vi "Force_Sensing2.vi"() -> ()   [LabVIEW 2014]
uses:
  <vilib>/Analysis/Matrix/Datatypes/RealMatrix.ctl
  <vilib>/Analysis/3filter.llb/Filter Passband Type.ctl
  <vilib>/Analysis/baseanly.llb/Real A x B.vi
  <vilib>/Analysis/_algsub.llb/Real PseudoInverse Matrix.vi
  <vilib>/Analysis/_algsub.llb/Real Vector Norm.vi
  <vilib>/Analysis/Matrix/Numeric/Conversions/Array To Matrix - RA2.vi
  <vilib>/Analysis/Matrix/Numeric/Subtract/Subtract - RM,RM.vi
  <vilib>/Utility/file.llb/Write To Spreadsheet File (string).vi
  <vilib>/Analysis/NI_AALPro.lvlib
  <vilib>/Analysis/NI_AALBase.lvlib
  <vilib>/Analysis/Matrix/NI_Matrix.lvlib
  <vilib>/ptbypt/NI_PtbyPt.lvlib
panel:
  out "Product":dbl(slide) scale=-1.0..1.0
  out "Filtered Force":T1
  out "Filtered Position":T1
  out "F_TM":T1
  in  "Puncture false":bool
  out "FilteredForceDerivative":dbl(slide) caption="Force Derivative"
  in  "stop":bool
  in  "low cutoff freq: fl":dbl=0.5 format="%0.3f"
  in  "high cutoff freq: fh":dbl=100.0 format="%0.3f"
  in  "sampling freq: fs":dbl=15.0 format="%0.2f"
  out "Puncture":bool
  out "Tip position in Tracker coordinates [microns]":T1
  out "Tip force in Tracker coordinates [mN]":T1
  in  "dFthreshold":dbl=-0.1
  in  "Update":bool
  out "dF":dbl format="%.1f"
  out "Filtered dF":dbl format="%.1f"
  in  "Force Scaling Factor":dbl=1.0
  in  "Record Switch":bool
  in  "file path (dialog if empty)":path=path "C:/Users/MICRON/Desktop/Hold_repeat/XY1"
  in  "Audio Switch":bool
  out "Measured Tip Forces [mN]":u8(slide) scale=0.0..10.0
  in  "Plot Switch":bool
  out "Ftotal [mN]":dbl
  out "Fy [mN]":dbl
  out "Fx [mN]":dbl
  in  "sm130 IP Address":string="192.168.1.126"
  in  "Rebias":bool
  out "Active Calibration Matrix":dbl[][](array[numeric])
  in  "Select Your Tool":T2(radio)=enum."2 DOF MicroNeedle CMU"
  out "Shift 3":dbl
  out "Shift 2":dbl
  out "Shift 1":dbl
  out "Channel 3":dbl format="%.3g"
  out "Channel 2":dbl format="%.3g"
  out "Channel 1":dbl format="%#.3g"
  out "Average 3":dbl format="%.3g"
  out "Average 2":dbl format="%.3g"
  out "Average 1":dbl format="%.3g"
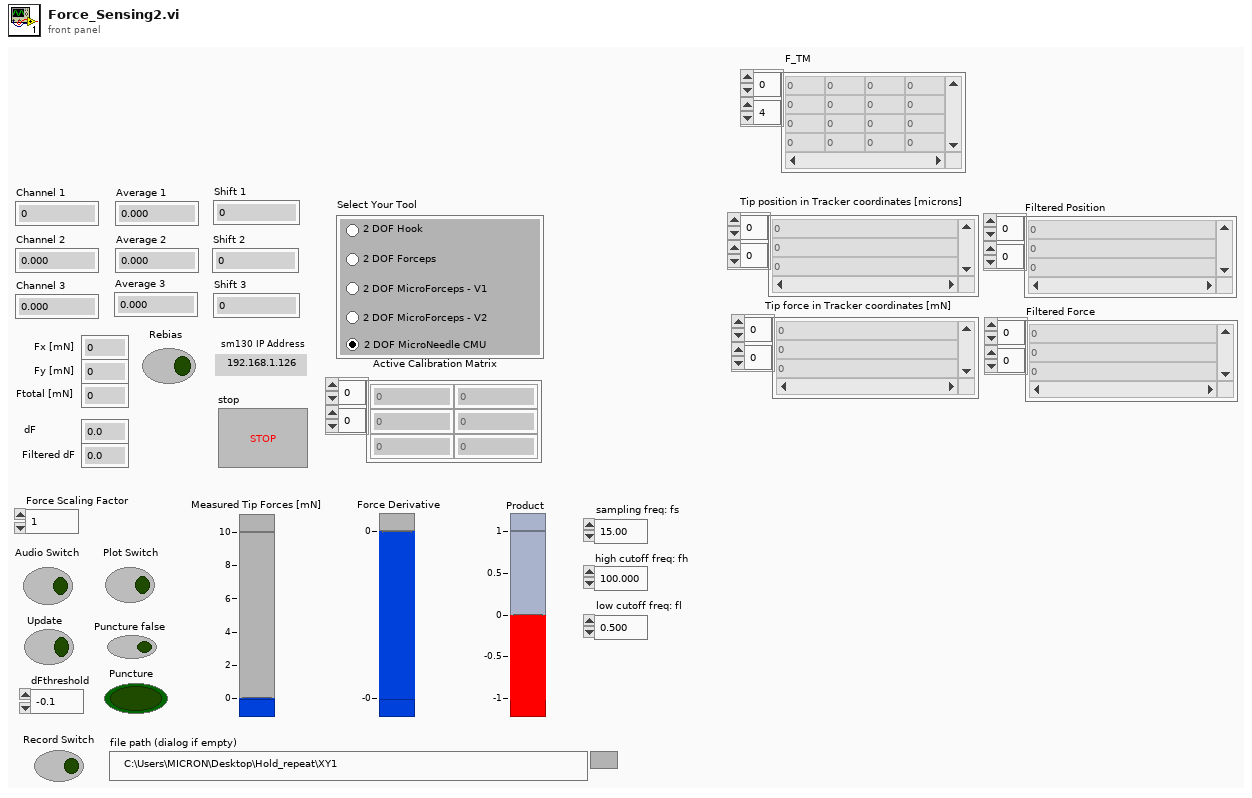
[diagram p1: front panel]
types:
  T1 = typedef "NI_Matrix.lvlib/RealMatrix.ctl" = dbl[][]
  T2 = enum32{"2 DOF Hook", "2 DOF Forceps", "2 DOF MicroForceps - V1", "2 DOF MicroForceps - V2", "2 DOF MicroNeedle CMU"}
  T3 = typedef "NI_AALBase.lvlib/Filter Passband Type.ctl" = enum32{"Lowpass", "Highpass", "Bandpass", "Bandstop"}
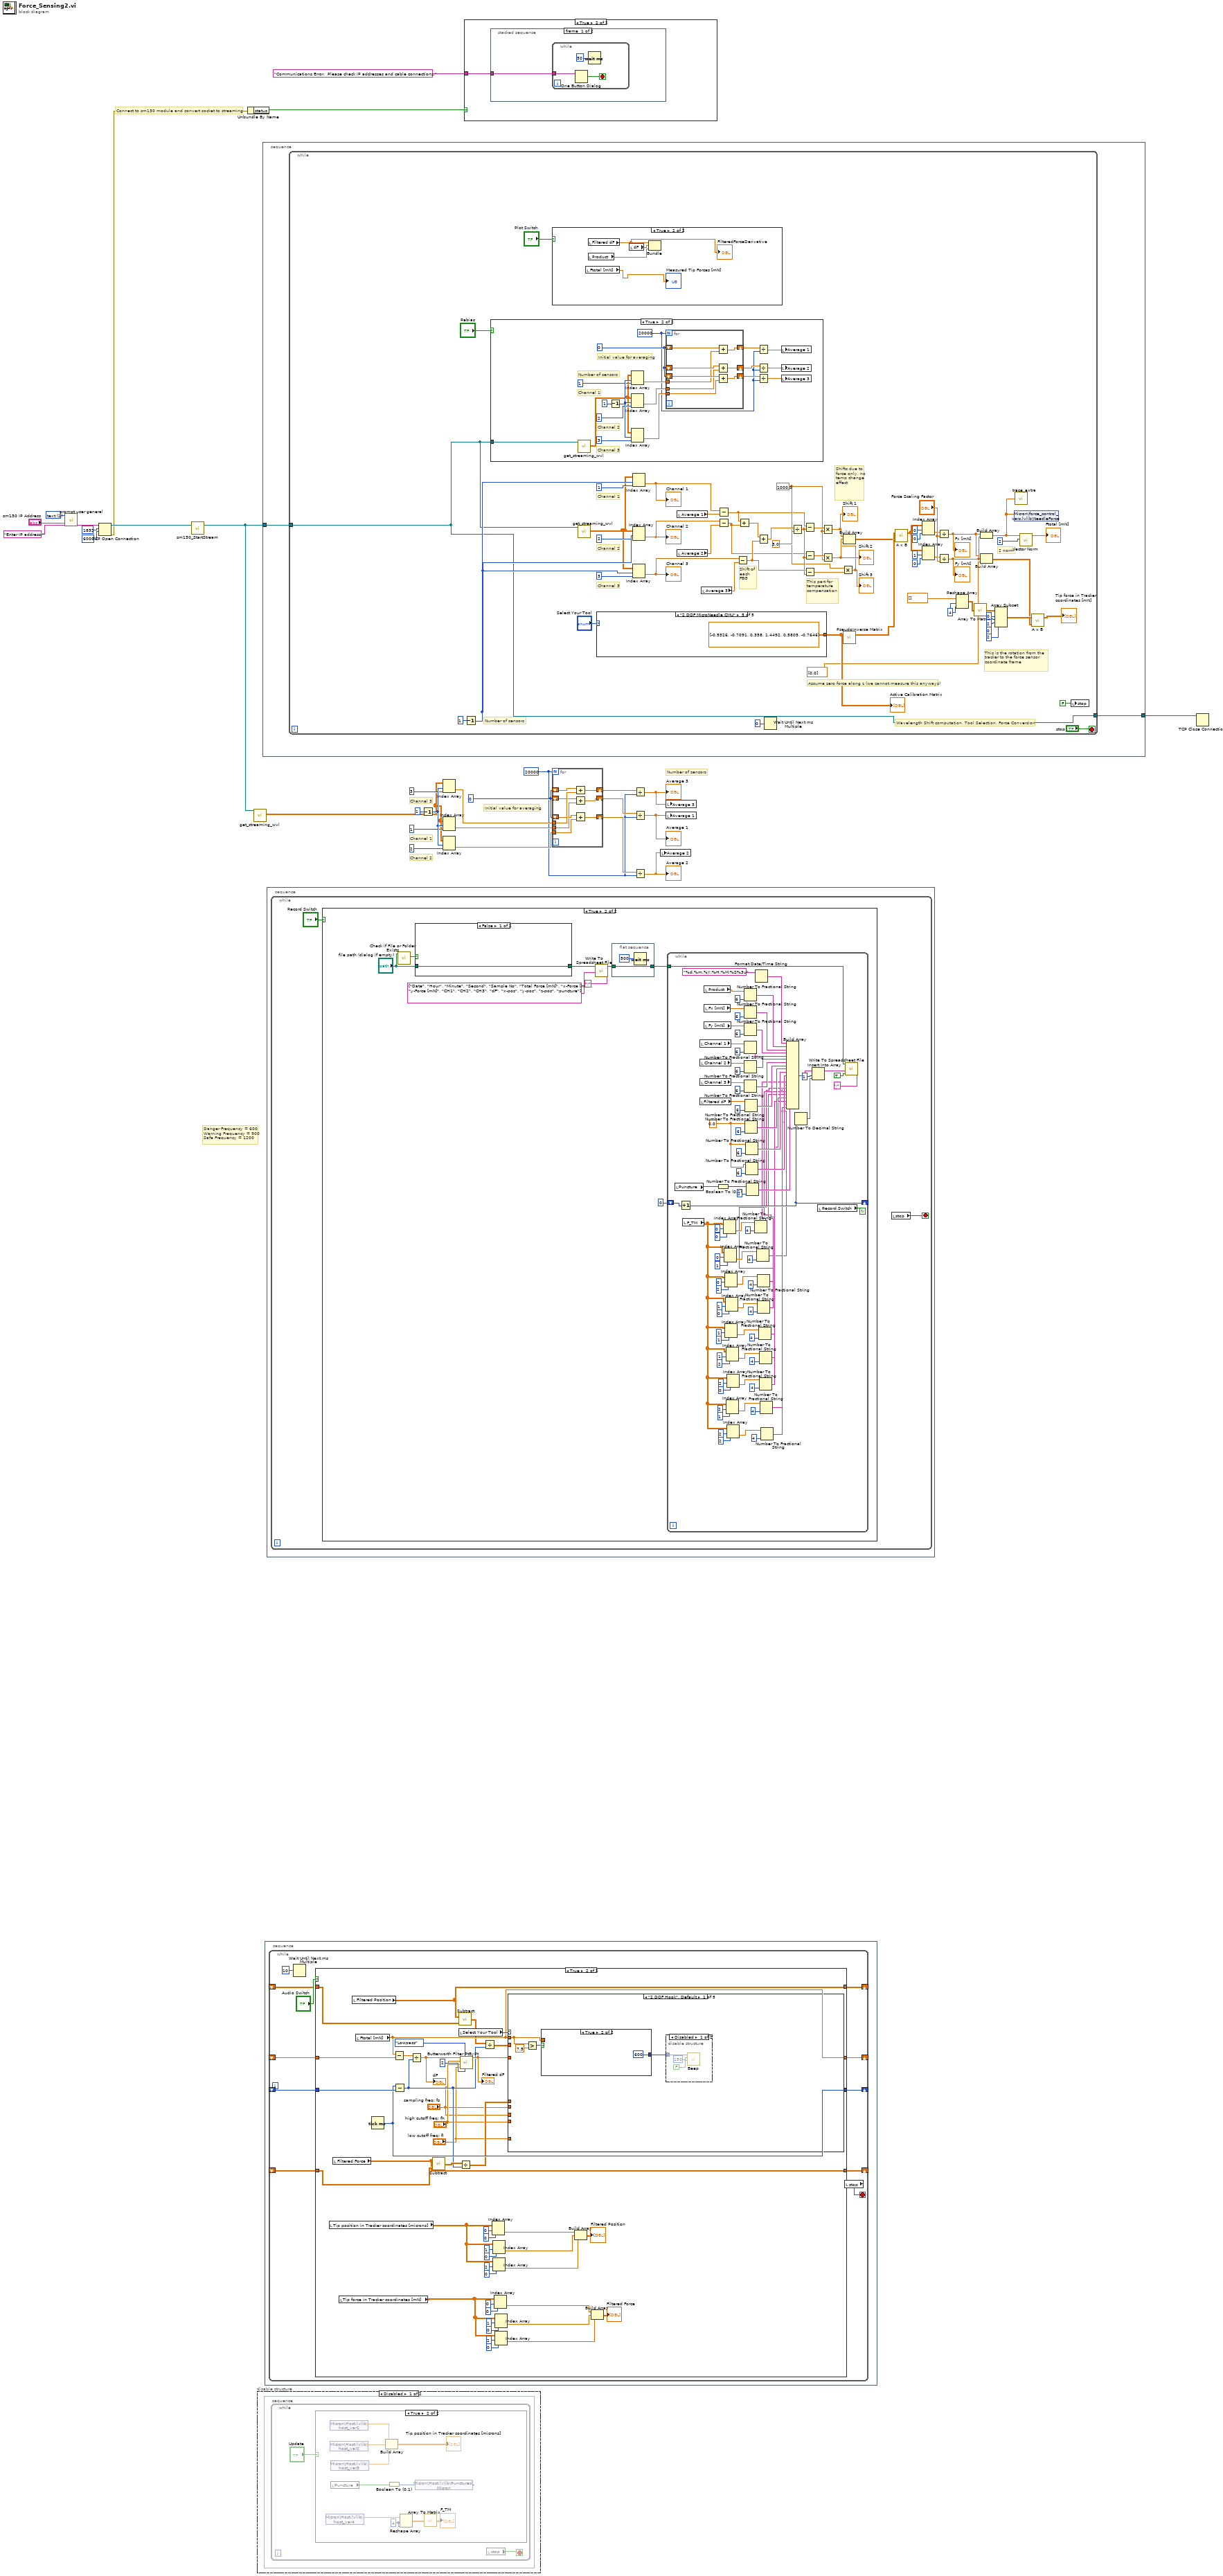
[diagram p0: block diagram]
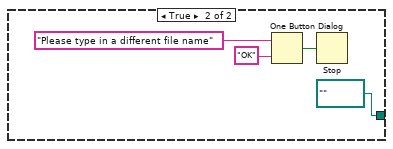
[diagram p5: hidden frame]
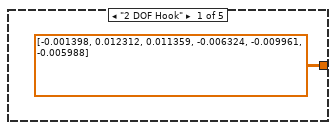
[diagram p8: hidden frame]
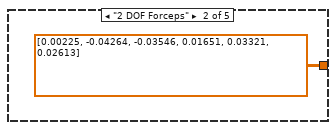
[diagram p9: hidden frame]
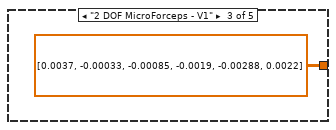
[diagram p10: hidden frame]
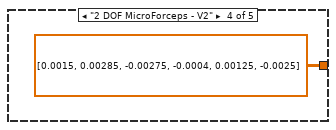
[diagram p11: hidden frame]
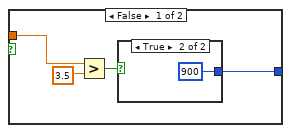
[diagram p14: hidden frame]
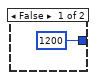
[diagram p15: hidden frame]
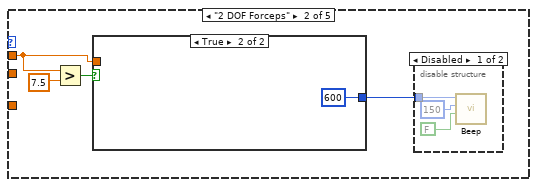
[diagram p16: hidden frame]
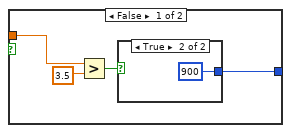
[diagram p18: hidden frame]
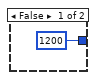
[diagram p19: hidden frame]
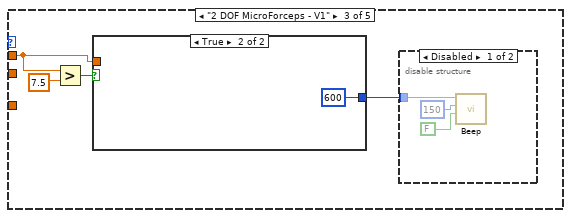
[diagram p20: hidden frame]
diagram:
  w4 = 20000
  w5 = 0
  w26 = u16 1 items=["numeric", "text"] ("control type")
  # "Danger Frequency = 600\nWarning Frequency = 900\nSafe Frequency = 1200"
  # "Initial value for averaging"
  # "Channel 3"
  # "Channel 2"
  # "Channel 1"
  # "Number of sensors"
  # "Connect to sm130 module and convert socket to streaming"
  n1 = call "prompt user general.vi"("control type"=w26, "text default"="sm130 IP Address", "message to display"="Enter IP address.") -> ("Text output"=w20:string)  [unwired: 11 in, 1 out]
  n2 = TCP Open Connection(address=w20, remote port or service name=u16 1852 ("remote port"), timeout ms (60000)=6000) -> (connection ID=w25:refnum<k5>, error out=w22:errorcluster)  [unwired: 2 in]
  n3 = call "sm130_StartStream.vi"("Connection ID In"=w25) -> ("Stream ID Out"=w28:refnum<k5>)  [unwired: 1 in, 1 out]
  n4 = Unbundle By Name(w22) -> ("status"=w21:bool)
  n5 = call "get_streaming_wvl.vi"("Stream ID Out"=w28) -> ("Array"=w12:dbl[][])  [unwired: 9 in, 1 out]
  n6 = disable-structure shown="Disabled" {
    frame Disabled {
      n7 = stacked-sequence {
        frame #0 {
          n8 = while {
            stop <- w30 stop-if-true
            n9 = case shown="True" "Update" {
              frame False {
              }
              frame True {
                w35 = 4 ("dimension size")
                n10 = shared-variable "Micron\\Host.lvlib\\host_var4"() -> (w32:dbl[])  [unwired: 1 in, 1 out]
                n11 = shared-variable "Micron\\Host.lvlib\\host_var1"() -> (w40:dbl)  [unwired: 1 in, 1 out]
                n12 = shared-variable "Micron\\Host.lvlib\\host_var2"() -> (w39:dbl)  [unwired: 1 in, 1 out]
                n13 = shared-variable "Micron\\Host.lvlib\\host_var3"() -> (w38:dbl)  [unwired: 1 in, 1 out]
                n14 = local read "Puncture"() -> (w37:bool)
                n15 = Build Array ("Build Matrix")(w40, w39, w38) -> (→"Tip position in Tracker coordinates [microns]":T1)
                n16 = Boolean To (0,1)(Boolean=w37) -> (0, 1=w36:i16)
                n17 = Reshape Array(w32, w35, w35) -> (w34:dbl[][])
                n18 = shared-variable "Micron\\Host.lvlib\\Punctured_Micron"(w36) -> ()  [unwired: 1 in, 1 out]
                n19 = call-poly <vilib>:"Array To Matrix.vi"("Real 2D Array"=w34) -> ("Real Matrix"=→"F_TM":T1)
              }
            }
            n20 = local read "stop"() -> (w30:bool)
          }
        }
      }
    }
    frame Enabled {
    }
  }
  n21 = stacked-sequence {
    tunnel: w28 -> [w43]
    tunnel: [w42] -> w29
    frame #0 {
      n22 = while {
        tunnel: [w93] -> w42
        tunnel: w43 -> [w93]
        stop <- "stop" stop-if-true
        w52 = 1000.0 ("y")
        w66 = 4 ("dimension size")
        # "Shifts due to force only, no temp change effect"
        # "Shift of each FBG"
        # "This part for temperature compensation"
        # "Assume zero force along z (we cannot measure this anyways)"
        # "This is the rotation from the tracker to the force sensor coordinate frame"
        # "2 norm"
        # "Wavelength Shift computation, Tool Selection, Force Conversion"
        # "Channel 3"
        # "Channel 2"
        # "Channel 1"
        # "Number of sensors"
        n23 = Decrement(x=1) -> (x-1=w103:i32)
        n24 = case shown="True" "Rebias" {
          tunnel: w93 -> [_ w126]
          frame False {
          }
          frame True {
            w113 = 0
            w112 = 20000
            # "Initial value for averaging"
            # "Channel 3"
            # "Channel 2"
            # "Channel 1"
            # "Number of sensors"
            n25 = call "get_streaming_wvl.vi"("Stream ID Out"=w126) -> ("Array"=w120:dbl[][])  [unwired: 9 in, 1 out]
            n26 = Decrement(x=1) -> (x-1=w124:i32)
            n27 = Index Array(array=w120, index (row)=w124, index (col)=1) -> (element=w117:dbl)
            n28 = Index Array(array=w120, index (row)=w124, index (col)=2) -> (element=w118:dbl)
            n29 = Index Array(array=w120, index (row)=w124, index (col)=3) -> (element=w119:dbl)
            n30 = for {
              N: w112 -> [_]
              shift-right: [w129] -> w116
              shift-left: w113 -> [w128]
              shift-right: [w130] -> w115
              shift-left: w113 -> [w131]
              shift-right: [w135] -> w114
              shift-left: w113 -> [w133]
              tunnel: w119 -> [w134]
              tunnel: w118 -> [w132]
              tunnel: w117 -> [w127]
              n31 = Add(x=w128, y=w127) -> (x+y=w129:dbl)
              n32 = Add(x=w131, y=w132) -> (x+y=w130:dbl)
              n33 = Add(x=w133, y=w134) -> (x+y=w135:dbl)
            }
            n34 = Divide(x=w116, y=w112) -> (x/y=w111:dbl)
            n35 = Divide(x=w115, y=w112) -> (x/y=w110:dbl)
            n36 = Divide(x=w114, y=w112) -> (x/y=w109:dbl)
            n37 = local write "Average 1"(w111) -> ()
            n38 = local write "Average 2"(w110) -> ()
            n39 = local write "Average 3"(w109) -> ()
          }
        }
        n40 = case shown="True" "Plot Switch" {
          frame False {
          }
          frame True {
            n41 = local read "Ftotal [mN]"() -> (→"Measured Tip Forces [mN]":dbl)
            n42 = local read "Filtered dF"() -> (w105:dbl)
            "FilteredForceDerivative" <- w105
            n43 = local read "Product"() -> (w107:dbl)
            n44 = local read "dF"() -> (w108:dbl)
            n45 = Bundle("Filtered dF"=w105, "dF"=w108, "Product"=w107) -> ()  [unwired: 1 in, 1 out]
          }
        }
        n46 = call "get_streaming_wvl.vi"("Stream ID Out"=w93) -> ("Array"=w99:dbl[][])  [unwired: 9 in, 1 out]
        n47 = case shown="\"2 DOF MicroNeedle CMU\"" "Select Your Tool" {
          tunnel: [T1 [[-0.001398, 0.012312], [0.011359, -0.006324], [-0.009961, -0.005988]] ("output matrix") T1 [[0.00225, -0.04264], [-0.03546, 0.01651], [0.03321, 0.02613]] ("output matrix") T1 [[0.0037, -0.00033], [-0.00085, -0.0019], [-0.00288, 0.0022]] ("output matrix") T1 [[0.0015, 0.00285], [-0.00275, -0.0004], [0.00125, -0.0025]] ("output matrix") T1 [[-0.9326, -0.7091], [0.358, 1.4492], [0.5805, -0.7646]] ("output matrix")] -> w91
          frame "2 DOF Hook" {
          }
          frame "2 DOF Forceps" {
          }
          frame "2 DOF MicroForceps - V1" {
          }
          frame "2 DOF MicroForceps - V2" {
          }
          frame "2 DOF MicroNeedle CMU" {
          }
        }
        "Active Calibration Matrix" <- w91
        n48 = Index Array(array=w99, index (row)=w103, index (col)=1) -> (element=w71:dbl)
        "Channel 1" <- w71
        n49 = Index Array(array=w99, index (row)=w103, index (col)=2) -> (element=w73:dbl)
        "Channel 2" <- w73
        n50 = Index Array(array=w99, index (row)=w103, index (col)=3) -> (element=w72:dbl)
        "Channel 3" <- w72
        n51 = local read "Average 1"() -> (w95:dbl)
        n52 = local read "Average 2"() -> (w94:dbl)
        n53 = local read "Average 3"() -> (w96:dbl)
        n54 = Subtract(x=w71, y=w95) -> (x-y=w46:dbl)
        n55 = Subtract(x=w73, y=w94) -> (x-y=w47:dbl)
        n56 = Subtract(x=w72, y=w96) -> (x-y=w76:dbl)
        n57 = Add(x=w46, y=w47) -> (x+y=w48:dbl)
        n58 = Add(x=w48, y=w76) -> (x+y=w79:dbl)
        n59 = Wait Until Next ms Multiple(millisecond multiple=0) -> ()  [unwired: 1 out]
        n60 = Divide(x=w79, y=3.0) -> (x/y=w77:dbl)
        n61 = Subtract(x=w46, y=w77) -> (x-y=w55:dbl)
        n62 = Subtract(x=w47, y=w77) -> (x-y=w53:dbl)
        n63 = Subtract(x=w76, y=w77) -> (x-y=w54:dbl)
        n64 = Multiply(x=w55, y=w52) -> (x*y=w45:dbl)
        "Shift 1" <- w45
        n65 = Multiply(x=w53, y=w52) -> (x*y=w51:dbl)
        "Shift 2" <- w51
        n66 = Multiply(x=w52, y=w54) -> (x*y=w50:dbl)
        "Shift 3" <- w50
        n67 = Build Array ("Build Matrix")(w45, w51, w50) -> (w97:T1)
        n68 = call-poly <vilib>:"PseudoInverse Matrix.vi"("Input Matrix"=w91) -> ("PseudoInverse Matrix"=w98:T1)  [unwired: 1 in, 1 out]
        n69 = call-poly <vilib>:"A x B.vi"("B"=w97, "A"=w98) -> ("A x B"=w89:T1)  [unwired: 1 out]
        n70 = Index Array(array=w89, index (row)=0, index (col)=0 ("index (row)")) -> (element=w70:dbl)
        n71 = Index Array(array=w89, index (row)=1, index (col)=0 ("index (row)")) -> (element=w69:dbl)
        n72 = Divide(x=w70, y="Force Scaling Factor") -> (x/y=w49:dbl)
        "Fx [mN]" <- w49
        n73 = Divide(x=w69, y="Force Scaling Factor") -> (x/y=w74:dbl)
        "Fy [mN]" <- w74
        n74 = Reshape Array(dbl[] [] ("array"), w66, w66) -> (w65:dbl[][])
        n75 = call-poly <vilib>:"Array To Matrix.vi"("Real 2D Array"=w65) -> ("Real Matrix"=w64:T1)
        n76 = Build Array(w49, w74) -> (w44:dbl[])
        n77 = Build Array ("Build Matrix")(w49, w74, dbl[] [0.0] ("element")) -> (w62:T1)
        n78 = Array Subset(array=w64, index (row)=0 ("row 1"), length (row)=2 ("row N"), index (col)=0 ("column 1"), length (col)=2 ("column N")) -> (w63:T1)
        n79 = shared-variable "Micron\\force_control_vars.lvlib\\NeedleForce"(w44) -> ()  [unwired: 1 in, 1 out]
        n80 = call "trace_extra.vi"("Extra trace data"=w44) -> ()  [unwired: 1 in]
        n81 = call-poly <vilib>:"Vector Norm.vi"("norm type"=2, "Input Vector"=w44) -> ("norm"=→"Ftotal [mN]":dbl)  [unwired: 8 in, 1 out]
        n82 = call-poly <vilib>:"A x B.vi"("B"=w62, "A"=w63) -> ("A x B"=→"Tip force in Tracker coordinates [mN]":T1)  [unwired: 1 out]
        n83 = local write "stop"(FALSE) -> ()
      }
    }
  }
  n84 = stacked-sequence {
    frame #0 {
      n85 = while {
        shift-right: [w148] -> _
        shift-left: _ -> [w149]
        shift-right: [w146] -> _
        shift-left: _ -> [w147]
        shift-right: [w145] -> _
        shift-left: _ -> [w144]
        shift-right: [w142] -> _
        shift-left: _ -> [w143]
        stop <- w141 stop-if-true
        n86 = Wait Until Next ms Multiple(millisecond multiple=10) -> ()  [unwired: 1 out]
        n87 = case shown="True" "Audio Switch" {
          tunnel: w149 -> [w155 w199]
          tunnel: [w155 w198] -> w148
          tunnel: w147 -> [w154 w196]
          tunnel: [w154 w192] -> w146
          tunnel: [w153 w165] -> w145
          tunnel: w144 -> [w153 w189]
          tunnel: w143 -> [w152 w185]
          tunnel: [w152 w177] -> w142
          frame False {
          }
          frame True {
            n88 = local read "Tip position in Tracker coordinates [microns]"() -> (w182:T1)
            n89 = local read "Filtered Force"() -> (w165:T1)
            n90 = local read "Tip force in Tracker coordinates [mN]"() -> (w167:T1)
            n91 = local read "Filtered Position"() -> (w177:T1)
            n92 = local read "Ftotal [mN]"() -> (w192:dbl)
            n93 = Tick Count (ms)() -> (millisecond timer value=w198:u32)
            n94 = Subtract(x=w192, y=w196) -> (x-y=w197:dbl)
            n95 = Subtract(x=w198, y=w199) -> (x-y=w187:u32)
            n96 = Divide(x=w197, y=w187) -> (x/y=w183:dbl)
            "dF" <- w183
            n97 = call-poly <vilib>:"Subtract.vi"("Real Matrix B"=w189, "Real Matrix A"=w165) -> ("A - B"=w190:T1)
            n98 = local read "Select Your Tool"() -> (w193:T2)
            n99 = call-poly <vilib>:"Subtract.vi"("Real Matrix B"=w185, "Real Matrix A"=w177) -> ("A - B"=w184:T1)
            n100 = Divide(x=w190, y=w187) -> (x/y=w188:T1)
            n101 = call <vilib>:"Butterworth Filter PtByPt.vi"("order"=2, "filter type"=Filter_Passband_Type."Lowpass", "low cutoff freq: fl"="low cutoff freq: fl", "high cutoff freq: fh"="high cutoff freq: fh", "sampling freq: fs"="sampling freq: fs", "x"=w183) -> ("Filtered x"=w191:dbl)  [unwired: 3 in, 1 out]
            "Filtered dF" <- w191
            n102 = Divide(x=w184, y=w187) -> (x/y=w186:T1)
            n103 = Index Array(array=w182, index (row)=0, index (col)=0 ("disabled index (col)")) -> (element=w164:dbl)
            n104 = Index Array(array=w182, index (row)=1, index (col)=0 ("disabled index (col)")) -> (element=w163:dbl)
            n105 = Index Array(array=w182, index (row)=2, index (col)=0 ("disabled index (col)")) -> (element=w162:dbl)
            n106 = Index Array(array=w167, index (row)=0, index (col)=0 ("disabled index (col)")) -> (element=w161:dbl)
            n107 = Index Array(array=w167, index (row)=1, index (col)=0 ("disabled index (col)")) -> (element=w160:dbl)
            n108 = Index Array(array=w167, index (row)=2, index (col)=0 ("disabled index (col)")) -> (element=w159:dbl)
            n109 = case shown="\"2 DOF Hook\", Default" w193 {
              tunnel: w192 -> [w201 w215 w229 w243 _]
              tunnel: w191 -> [_ _ _ _ w263]
              tunnel: w188 -> [_ _ _ _ w266]
              tunnel: w186 -> [_ _ _ _ w264]
              tunnel: "sampling freq: fs" -> [_ _ _ _ _]
              tunnel: "high cutoff freq: fh" -> [_ _ _ _ w257]
              tunnel: "low cutoff freq: fl" -> [_ _ _ _ w256]
              tunnel: "sampling freq: fs" -> [_ _ _ _ w258]
              frame "2 DOF Hook", Default {
                n110 = Greater?(x=w201, y=7.5) -> (0:w203:bool)
                n111 = case shown="True" w203 {
                  tunnel: [w208 600] -> w202
                  tunnel: w201 -> [w210 _]
                  frame False {
                    n112 = Greater?(x=w210, y=3.5) -> (0:w209:bool)
                    n113 = case shown="True" w209 {
                      tunnel: [1200 900] -> w208
                      frame False {
                      }
                      frame True {
                      }
                    }
                  }
                  frame True {
                  }
                }
                n114 = disable-structure shown="Disabled" {
                  disable-tunnel: w202 -> [w206 _]
                  frame Disabled {
                    n115 = call <vilib>:"Beep.vi"("use system alert? (T)"=FALSE, "duration (msec)"=150, "frequency (Hz)"=w206) -> ()  [unwired: 9 in]
                  }
                  frame Enabled {
                  }
                }
              }
              frame "2 DOF Forceps" {
                n116 = Greater?(x=w215, y=7.5) -> (0:w217:bool)
                n117 = case shown="True" w217 {
                  tunnel: [w222 600] -> w216
                  tunnel: w215 -> [w224 _]
                  frame False {
                    n118 = Greater?(x=w224, y=3.5) -> (0:w223:bool)
                    n119 = case shown="True" w223 {
                      tunnel: [1200 900] -> w222
                      frame False {
                      }
                      frame True {
                      }
                    }
                  }
                  frame True {
                  }
                }
                n120 = disable-structure shown="Disabled" {
                  disable-tunnel: w216 -> [w220 _]
                  frame Disabled {
                    n121 = call <vilib>:"Beep.vi"("use system alert? (T)"=FALSE, "duration (msec)"=150, "frequency (Hz)"=w220) -> ()  [unwired: 9 in]
                  }
                  frame Enabled {
                  }
                }
              }
              frame "2 DOF MicroForceps - V1" {
                n122 = Greater?(x=w229, y=7.5) -> (0:w231:bool)
                n123 = case shown="True" w231 {
                  tunnel: [w236 600] -> w230
                  tunnel: w229 -> [w238 _]
                  frame False {
                    n124 = Greater?(x=w238, y=3.5) -> (0:w237:bool)
                    n125 = case shown="True" w237 {
                      tunnel: [1200 900] -> w236
                      frame False {
                      }
                      frame True {
                      }
                    }
                  }
                  frame True {
                  }
                }
                n126 = disable-structure shown="Disabled" {
                  disable-tunnel: w230 -> [w234 _]
                  frame Disabled {
                    n127 = call <vilib>:"Beep.vi"("use system alert? (T)"=FALSE, "duration (msec)"=150, "frequency (Hz)"=w234) -> ()  [unwired: 9 in]
                  }
                  frame Enabled {
                  }
                }
              }
              frame "2 DOF MicroForceps - V2" {
                n128 = Greater?(x=w243, y=7.5) -> (0:w245:bool)
                n129 = case shown="True" w245 {
                  tunnel: [w250 600] -> w244
                  tunnel: w243 -> [w252 _]
                  frame False {
                    n130 = Greater?(x=w252, y=3.5) -> (0:w251:bool)
                    n131 = case shown="True" w251 {
                      tunnel: [1200 900] -> w250
                      frame False {
                      }
                      frame True {
                      }
                    }
                  }
                  frame True {
                  }
                }
                n132 = disable-structure shown="Disabled" {
                  disable-tunnel: w244 -> [w248 _]
                  frame Disabled {
                    n133 = call <vilib>:"Beep.vi"("use system alert? (T)"=FALSE, "duration (msec)"=150, "frequency (Hz)"=w248) -> ()  [unwired: 9 in]
                  }
                  frame Enabled {
                  }
                }
              }
              frame "2 DOF MicroNeedle CMU" {
                # "If the force is dropping, although the position is increasing, then give an alarm"
                n134 = Transpose Matrix(1:w264) -> (0:w267:T1)
                n135 = call-poly <vilib>:"A x B.vi"("B"=w266, "A"=w267) -> ("A x B"=w265:T1)  [unwired: 1 out]
                n136 = Index Array(array=w265, index (row)=0, index (col)=0 ("index (row)")) -> (element=w260:dbl)
                n137 = Less?(x=w263, y="dFthreshold") -> (x < y?=w261:bool)
                n138 = call <vilib>:"Butterworth Filter PtByPt.vi"("low cutoff freq: fl"=w256, "high cutoff freq: fh"=w257, "sampling freq: fs"=w258, "x"=w260) -> ("Filtered x"=→"Product":dbl)  [unwired: 5 in, 1 out]
                n139 = case shown="True" "Puncture false" {
                  frame False {
                  }
                  frame True {
                    n140 = local write "Puncture"(FALSE ("Puncture")) -> ()
                  }
                }
                n141 = case shown="True" w261 {
                  frame False {
                  }
                  frame True {
                    n142 = disable-structure shown="Disabled" {
                      frame Disabled {
                        n143 = call <vilib>:"Beep.vi"("use system alert? (T)"=FALSE, "duration (msec)"=u32 150, "frequency (Hz)"=u32 600) -> ()  [unwired: 9 in]
                      }
                      frame Enabled {
                      }
                    }
                    "Puncture" <- TRUE ("Puncture")
                  }
                }
              }
            }
            n144 = Build Array(w164, w163, w162) -> (→"Filtered Position":T1)
            n145 = Build Array(w161, w160, w159) -> (→"Filtered Force":T1)
          }
        }
        n146 = local read "stop"() -> (w141:bool)
      }
    }
  }
  n147 = stacked-sequence {
    frame #0 {
      n148 = while {
        stop <- w276 stop-if-true
        n149 = case shown="True" "Record Switch" {
          frame False {
          }
          frame True {
            n150 = call <vilib>:"Check if File or Folder Exists.vi"("path"="file path (dialog if empty)") -> ("file or folder exists?"=w282:bool)  [unwired: 8 in, 2 out]
            n151 = case shown="False" w282 {
              tunnel: [w376 path "" ("file path (dialog if empty)")] -> w283
              tunnel: "file path (dialog if empty)" -> [w376 _]
              frame False {
              }
              frame True {
                n152 = One Button Dialog(message="Please type in a different file name", button name ("OK")="OK") -> (true=w378:bool)
                n153 = Stop(stop? (T)=w378) -> ()
              }
            }
            n154 = call-poly <vilib>:"Write To Spreadsheet File.vi"("delimiter (\\t)"=";" ("delimiter (\\t)"), "1D data"=string[] ["Date", "Hour", "Minute", "Second", "Sample No", "Total Force [mN]", "x-Force [mN]", "y-Force [mN]", "CH1", "CH2", "CH3", "dF", "x-pos", "y-pos", "z-pos", "puncture"], "file path (dialog if empty)"=w283) -> ("new file path (Not A Path if cancelled)"=w280:path)  [unwired: 5 in]
            n155 = flat-sequence {
              tunnel: [w381] -> w279
              tunnel: w280 -> [w381]
              frame #0 {
                n156 = Wait (ms)(milliseconds to wait=u32 500) -> ()  [unwired: 1 out]
              }
            }
            n157 = while {
              shift-right: [w368] -> _
              shift-left: 0 -> [w357]
              tunnel: w279 -> [w356]
              stop <- w349 continue-if-true
              w286 = 0.0 ("number")
              n158 = local read "Puncture"() -> (w335:bool)
              n159 = Increment(x=w357) -> (x+1=w368:i32)
              n160 = local read "F_TM"() -> (w314:T1)
              n161 = local read "Filtered dF"() -> (w348:dbl)
              n162 = local read "Channel 1"() -> (w351:dbl)
              n163 = local read "Channel 2"() -> (w352:dbl)
              n164 = local read "Channel 3"() -> (w350:dbl)
              n165 = local read "Product"() -> (w364:dbl)
              n166 = local read "Fx [mN]"() -> (w361:dbl)
              n167 = local read "Fy [mN]"() -> (w360:dbl)
              n168 = Boolean To (0,1)(Boolean=w335) -> (0, 1=w334:i16)
              n169 = Index Array(array=w314, index (row)=0, index (col)=0) -> (element=w304:dbl)
              n170 = Index Array(array=w314, index (row)=0, index (col)=1) -> (element=w303:dbl)
              n171 = Index Array(array=w314, index (row)=0, index (col)=2) -> (element=w302:dbl)
              n172 = Index Array(array=w314, index (row)=1, index (col)=1) -> (element=w300:dbl)
              n173 = Index Array(array=w314, index (row)=1, index (col)=0) -> (element=w301:dbl)
              n174 = Index Array(array=w314, index (row)=1, index (col)=2) -> (element=w299:dbl)
              n175 = Index Array(array=w314, index (row)=2, index (col)=1) -> (element=w297:dbl)
              n176 = Index Array(array=w314, index (row)=2, index (col)=0) -> (element=w298:dbl)
              n177 = Index Array(array=w314, index (row)=2, index (col)=2) -> (element=w296:dbl)
              n178 = Number To Fractional String(number=w364, precision (6)=i16 6) -> (F-format string=w372:string)  [unwired: 2 in]
              n179 = Number To Fractional String(number=w361, precision (6)=i16 6) -> (F-format string=w359:string)  [unwired: 2 in]
              n180 = Number To Fractional String(number=w360, precision (6)=i16 6) -> (F-format string=w358:string)  [unwired: 2 in]
              n181 = Number To Fractional String(number=w351, precision (6)=i16 6) -> (F-format string=w346:string)  [unwired: 2 in]
              n182 = Number To Fractional String(number=w352, precision (6)=i16 6) -> (F-format string=w345:string)  [unwired: 2 in]
              n183 = Number To Fractional String(number=w350, precision (6)=i16 6) -> (F-format string=w344:string)  [unwired: 2 in]
              n184 = Number To Fractional String(number=w348, precision (6)=i16 6) -> (F-format string=w343:string)  [unwired: 2 in]
              n185 = Number To Fractional String(number=w286, precision (6)=i16 6) -> (F-format string=w339:string)  [unwired: 2 in]
              n186 = Number To Fractional String(number=w286, precision (6)=i16 6) -> (F-format string=w338:string)  [unwired: 2 in]
              n187 = Number To Fractional String(number=w286, precision (6)=i16 6) -> (F-format string=w337:string)  [unwired: 2 in]
              n188 = Number To Fractional String(number=w334, precision (6)=i16 2) -> (F-format string=w333:string)  [unwired: 2 in]
              n189 = Number To Fractional String(number=w304, precision (6)=i16 4) -> (F-format string=w287:string)  [unwired: 2 in]
              n190 = Format Date/Time String(time format string (%c)="%d.%m.%Y;%H;%M;%S%3u") -> (date/time string=w374:string)  [unwired: 2 in]
              n191 = Number To Fractional String(number=w303, precision (6)=i16 4) -> (F-format string=w288:string)  [unwired: 2 in]
              n192 = Number To Fractional String(number=w302, precision (6)=i16 4) -> (F-format string=w289:string)  [unwired: 2 in]
              n193 = Number To Fractional String(number=w301, precision (6)=i16 4) -> (F-format string=w290:string)  [unwired: 2 in]
              n194 = Number To Fractional String(number=w300, precision (6)=i16 4) -> (F-format string=w291:string)  [unwired: 2 in]
              n195 = Number To Fractional String(number=w299, precision (6)=i16 4) -> (F-format string=w292:string)  [unwired: 2 in]
              n196 = Number To Fractional String(number=w298, precision (6)=i16 4) -> (F-format string=w293:string)  [unwired: 2 in]
              n197 = Number To Fractional String(number=w297, precision (6)=i16 4) -> (F-format string=w294:string)  [unwired: 2 in]
              n198 = Number To Fractional String(number=w296, precision (6)=i16 4) -> (F-format string=w295:string)  [unwired: 2 in]
              n199 = Build Array(w374, w372, w359, w358, w346, w345, w344, w343, w339, w338, w337, w333, w287, w288, w289, w290, w291, w292, w293, w294, w295) -> (w371:string[])
              n200 = Number To Decimal String(number=w368) -> (decimal integer string=w369:string)  [unwired: 1 in]
              n201 = Insert Into Array(array=w371, index=1, new element=w369) -> (w367:string[])
              n202 = local read "Record Switch"() -> (w349:bool)
              n203 = call-poly <vilib>:"Write To Spreadsheet File.vi"("delimiter (\\t)"=";" ("delimiter (\\t)"), "append to file? (new file:F)"=TRUE, "1D data"=w367, "file path (dialog if empty)"=w356) -> ()  [unwired: 4 in, 1 out]
            }
          }
        }
        n204 = local read "stop"() -> (w276:bool)
      }
    }
  }
  n205 = Decrement(x=1) -> (x-1=w16:i32)
  n206 = Index Array(array=w12, index (row)=w16, index (col)=3) -> (element=w11:dbl)
  n207 = Index Array(array=w12, index (row)=w16, index (col)=1) -> (element=w9:dbl)
  n208 = Index Array(array=w12, index (row)=w16, index (col)=2) -> (element=w10:dbl)
  n209 = case shown="True" w21 {
    tunnel: "Communications Error.  Please check IP addresses and cable connections." ("message") -> [_ w383]
    frame False {
    }
    frame True {
      n210 = stacked-sequence {
        tunnel: w383 -> [w384 _]
        frame #0 {
          n211 = while {
            tunnel: w384 -> [w385]
            stop <- w387 stop-if-true
            n212 = One Button Dialog(message=w385) -> (true=w387:bool)  [unwired: 1 in]
            n213 = Wait (ms)(milliseconds to wait=u32 50) -> ()  [unwired: 1 out]
          }
        }
        frame #1 {
          n214 = Stop(stop? (T)=TRUE) -> ()
        }
      }
    }
  }
  n215 = for {
    N: w4 -> [_]
    shift-right: [w391] -> w8
    shift-left: w5 -> [w390]
    shift-right: [w392] -> w7
    shift-left: w5 -> [w393]
    shift-right: [w397] -> w6
    shift-left: w5 -> [w395]
    tunnel: w11 -> [w396]
    tunnel: w10 -> [w394]
    tunnel: w9 -> [w389]
    n216 = Add(x=w395, y=w396) -> (x+y=w397:dbl)
    n217 = Add(x=w390, y=w389) -> (x+y=w391:dbl)
    n218 = Add(x=w393, y=w394) -> (x+y=w392:dbl)
  }
  n219 = Divide(x=w6, y=w4) -> (x/y=w1:dbl)
  "Average 3" <- w1
  n220 = Divide(x=w8, y=w4) -> (x/y=w3:dbl)
  "Average 1" <- w3
  n221 = Divide(x=w7, y=w4) -> (x/y=w2:dbl)
  "Average 2" <- w2
  n222 = local write "Average 2"(w2) -> ()
  n223 = local write "Average 3"(w1) -> ()
  n224 = local write "Average 1"(w3) -> ()
  n225 = TCP Close Connection(connection ID=w29) -> ()  [unwired: 2 in, 2 out]
